vi "Write Notify idle.vi"(8 "error in (no error)":errorcluster, 10 "Notify idle":bool=TRUE, 11 "BaseDriver in":refnum<class "BaseDriver.lvclass">) -> (0 "error out":errorcluster, 3 "BaseDriver out":refnum<class "BaseDriver.lvclass">)   [LabVIEW 2013, in "BaseDriver.lvclass"]
doc: "If Notify Idle is set to TRUE, the driver will emit messages notifying the parent application when it becomes busy (has messages to send or are waiting for acknowledgements) and when it becomes Idle (no more messages to send or receive)"
uses:
  BaseDriver.lvclass
  BaseDriver.lvclass/BaseDriver.ctl
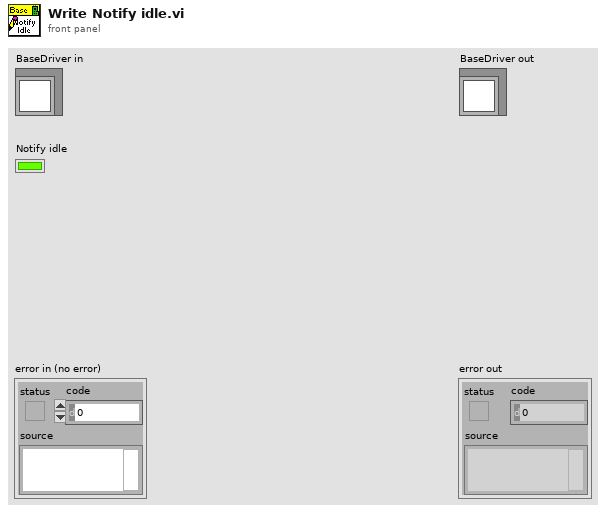
[diagram p1: front panel]
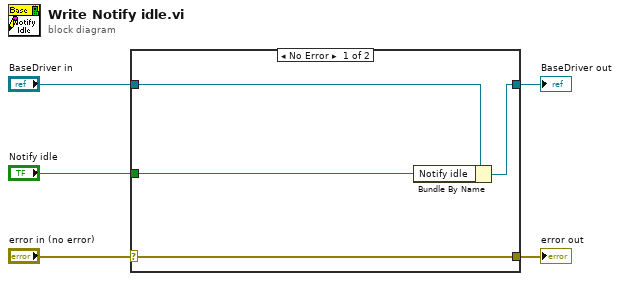
[diagram p0: block diagram]
diagram:
  n1 = case shown="No Error" "error in (no error)" {
    selector: "error in (no error)" -> [w9 w10]
    tunnel: [w9 w10] -> w4
    tunnel: [w7 w11] -> w2
    tunnel: "BaseDriver in" -> [w8 w11]
    tunnel: "Notify idle" -> [w6 _]
    frame No Error {
      n2 = Bundle By Name(cluster=w8, "Notify idle"=w6) -> (w7:refnum<class "BaseDriver.lvclass">)
    }
    frame Error {
    }
  }
  "error out" <- w4
  "BaseDriver out" <- w2
